vi "TextControlledInstrumUpdateControls.vi"(1 "Control To Index":T1(c390), 2 "Command Array":string[][](array[string]), 3 "timeout in ms (1000ms)":i32=1000, 9 "IO Queue":refnum<queue>) -> (8 "timed out?":bool)   [LabVIEW 2021]
uses:
  TextControlledInstrumIOQueuePacket.ctl
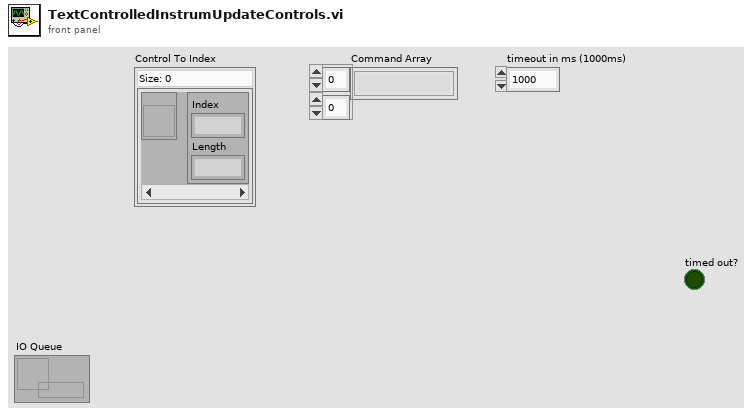
[diagram p1: front panel]
types:
  T1 = map{refnum<vi>, cluster{"Index":i32, "Length":i32}}
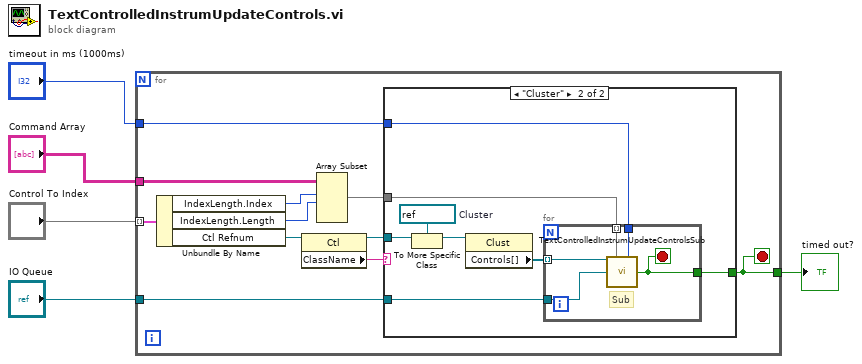
[diagram p0: block diagram]
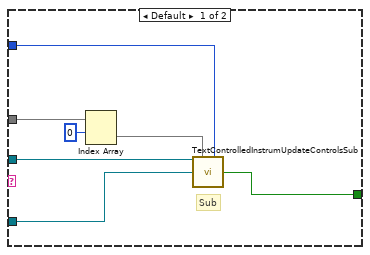
[diagram p2: hidden frame]
diagram:
  n1 = for {
    tunnel: "Control To Index" -> [w16] mode=indexing
    tunnel: "Command Array" -> [w15]
    tunnel: "timeout in ms (1000ms)" -> [w9]
    tunnel: "IO Queue" -> [w7]
    tunnel: [w6] -> w1
    stop <- w6 stop-if-true
    n2 = Unbundle By Name(w16) -> ("IndexLength.Index"=w14:i32, "IndexLength.Length"=w13:i32, "Ctl Refnum"=w12:refnum<vi>)
    n3 = property class="Ctl"(reference=w12) -> (reference out=w11:refnum<vi>, "ClassName"=w8:string)  [unwired: 1 in, 1 out]
    n4 = Array Subset(array=w15, index (row)=w14, length (row)=w13) -> (w10:string[][])  [unwired: 2 in]
    n5 = case shown="\"Cluster\"" w8 {
      tunnel: w11 -> [w23 w31]
      tunnel: w10 -> [w20 w26]
      tunnel: w9 -> [w22 w25]
      tunnel: w7 -> [w21 w27]
      tunnel: [w17 w24] -> w6
      frame Default {
        # "Sub"
        n6 = Index Array(array=w20, index (row)=0) -> (element=w18:string[])  [unwired: 1 in]
        n7 = call "TextControlledInstrumUpdateControlsSub.vi"("Control in"=w23, "SetGetCommands"=w18, "timeout in ms (1000ms)"=w22, "IO Queue"=w21) -> ("timed out?"=w17:bool)  [unwired: 11 in]
      }
      frame "Cluster" {
        w30 = refnum<vi> refnum  # Cluster
        n8 = To More Specific Class(target class=w30, reference=w31) -> (specific class reference=w29:refnum<vi>)  [unwired: 1 in, 1 out]
        n9 = property class="Clust"(reference=w29) -> ("Controls[]"=w28:refnum<vi>[])  [unwired: 1 in, 2 out]
        n10 = for {
          tunnel: w28 -> [w36] mode=indexing
          tunnel: w27 -> [w35]
          tunnel: w26 -> [w34] mode=indexing
          tunnel: w25 -> [w33]
          tunnel: [w32] -> w24
          stop <- w32 stop-if-true
          # "Sub"
          n11 = call "TextControlledInstrumUpdateControlsSub.vi"("Control in"=w36, "SetGetCommands"=w34, "timeout in ms (1000ms)"=w33, "IO Queue"=w35) -> ("timed out?"=w32:bool)  [unwired: 11 in]
        }
      }
    }
  }
  "timed out?" <- w1
